vi "Destination.vi"() -> ()   [LabVIEW 2014]
panel:
  out "Destination":string
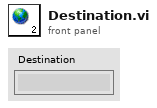
[diagram p1: front panel]
diagram:
